vi "roller.vi"   [LabVIEW 2011]
uses:
  roller_internal_state.ctl
  roller_user_state.ctl
  signals/Signal.ctl
  roller_output_state.ctl
  roller_globals.vi
types:
  T1 = typedef "roller_internal_state.ctl" = enum16{"idle", "bump", "full", "fire_intermediate", "fire_finish", "fire_entry", "fire_end", "fire_recover"}
  T2 = typedef "WPI_DigitalInputDevRef.ctl" = cluster{"DevStatus":errorcluster, "DIO Channel":T3, "Digital Module":T4}
  T3 = typedef "FPGA_DIOChannel.ctl" = enum8{"DIO 1", "DIO 2", "DIO 3", "DIO 4", "DIO 5", "DIO 6", "DIO 7", "DIO 8", "DIO 9", "DIO 10", "DIO 11", "DIO 12", "DIO 13", "DIO 14", "Invalid"}
  T4 = typedef "FPGA_TypedefDigitalModule.ctl" = enum16{"Digital Module 1", "Digital Module 2"}
  T5 = typedef "WPI_MotorControlDeviceRef.ctl" = cluster{"DeviceStatus":errorcluster, "Type":enum16{"PWM", "CAN"}, "PWM":cluster{"Digital Module":T4, "PWM Channel":T6, "DeadBand":T7}, "CAN":cluster{"Device Number":u8, "Control Mode":T8, "Semaphore":T9, "Max Vout":dbl}, "Invert":bool, "TransformRef":T10, "InvTransformRef":T10}
  T6 = typedef "FPGA_DIOPWMChannel.ctl" = enum8{"PWM 1", "PWM 2", "PWM 3", "PWM 4", "PWM 5", "PWM 6", "PWM 7", "PWM 8", "PWM 9", "PWM 10", "Invalid"}
  T7 = typedef "WPI_PWMDeadband.ctl" = cluster{"Name":string, "maxPositivePwm":i32, "minPositivePwm":i32, "centerPwm":i32, "maxNegativePwm":i32, "minNegativePwm":i32, "angularRange":u16}
  T8 = typedef "WPI_CANJaguar_ControlMode.ctl" = enum8{"Percent VBus", "Current", "Speed", "Position", "Voltage"}
  T9 = typedef "Semaphore RefNum" = refnum<k1>
  T10 = typedef "WPI_PWMTransform_ConPane.ctl" = refnum<vi>
  T11 = cluster{"DigitalInputDevRef":T2, "DigitalInputDevRef":T2, "DigitalInputDevRef":T2, "DigitalInputDevRef":T2, "DigitalInputDevRef":T2}
  T12 = typedef "roller_user_state.ctl" = enum16{"off", "collect", "blow", "force suck"}
  T13 = cluster{"roller internal state":T1, "roller user state":T12, "sws":cluster{"r_sw_b1":bool, "r_sw_b2":bool, "r_sw_b3":bool, "r_sw_gun":bool, "r_sw_low":bool}}
  T14 = enum16{"push_data", "write_joe_johnson", "write_roller", "write_drivetrain", "write_gun_fast", "write_gun_slow"}
  T15 = typedef "Signal.ctl" = enum16{"SIGFIRE", "SIGSTOPSCRIPT", "SIGSTARTGUN", "SIGSTOPGUN", "SIGDISABLED", "SIGENABLED", "SIGUDPTIMEOUT", "SIGNEWVISION_REMOTE", "SIGNEWVISION_LOCAL", "SIGSHOTFIRED", "SIGDOTRACK", "SIGDONTTRACK"}
  T16 = typedef "roller_output_state.ctl" = enum16{"off", "suck", "blow"}
  T17 = cluster{"r_sw_b1":bool, "r_sw_b2":bool, "r_sw_b3":bool, "r_sw_gun":bool, "r_sw_low":bool}
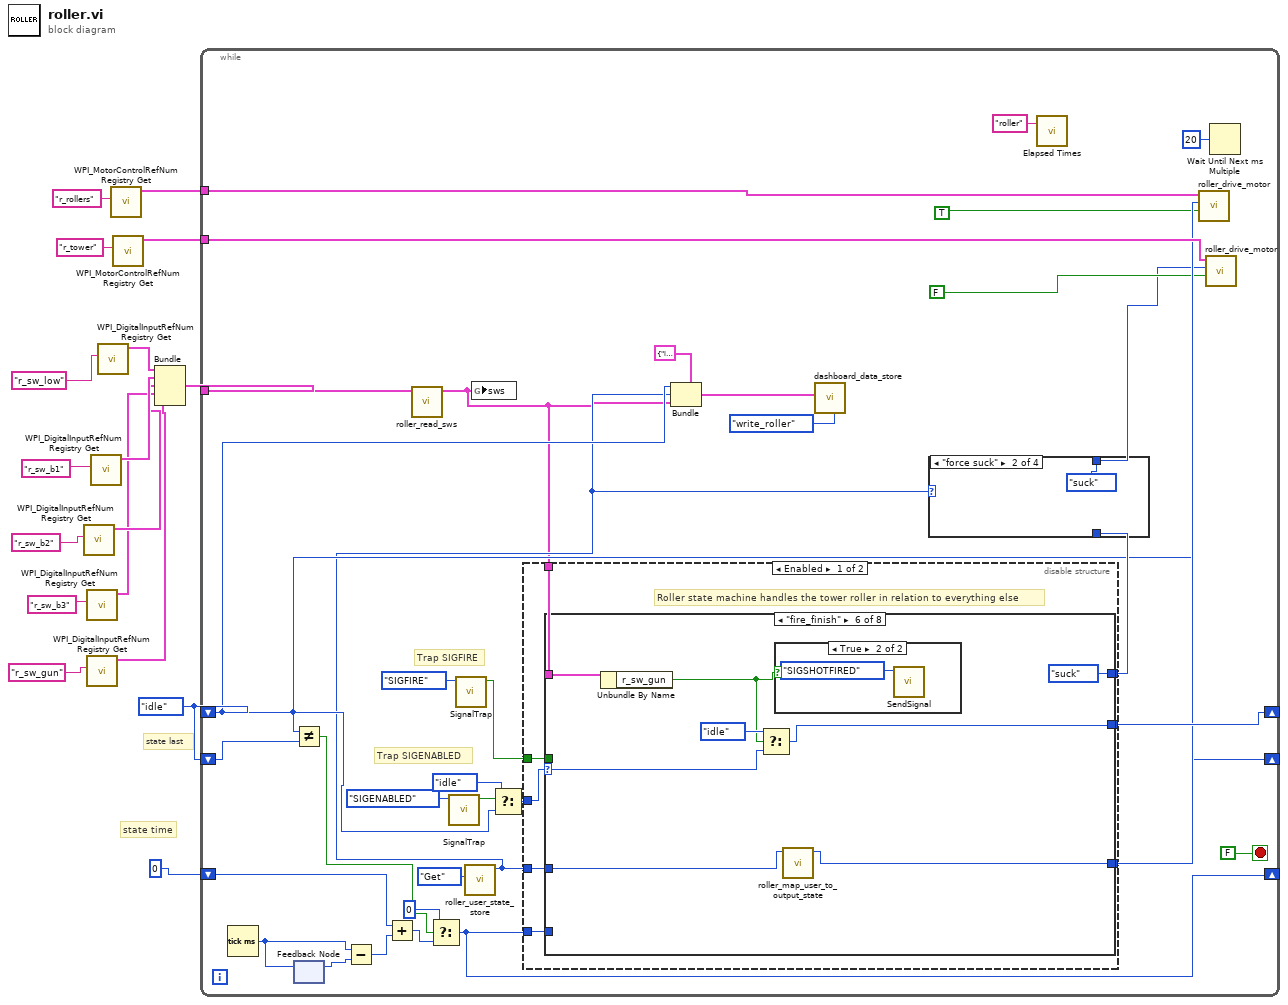
[diagram p0: block diagram]
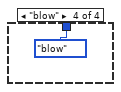
[diagram p4: hidden frame]
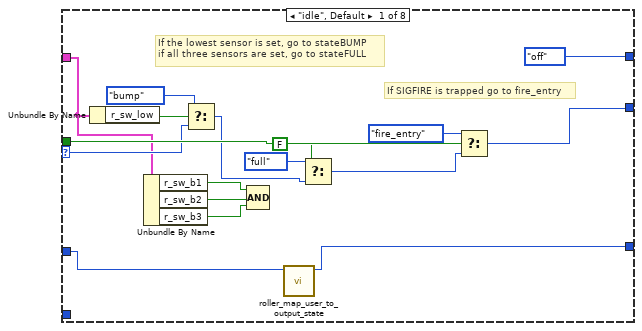
[diagram p5: hidden frame]
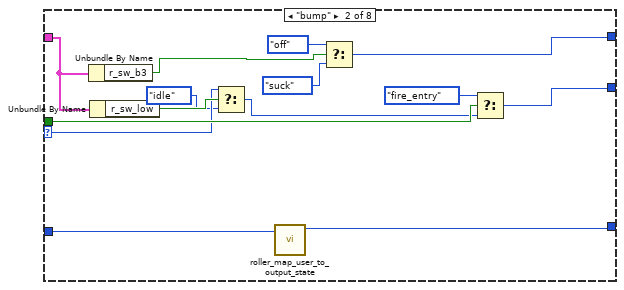
[diagram p6: hidden frame]
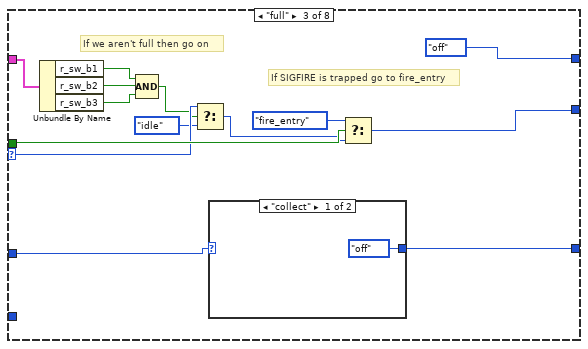
[diagram p7: hidden frame]
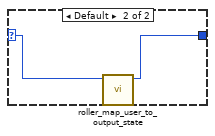
[diagram p8: hidden frame]
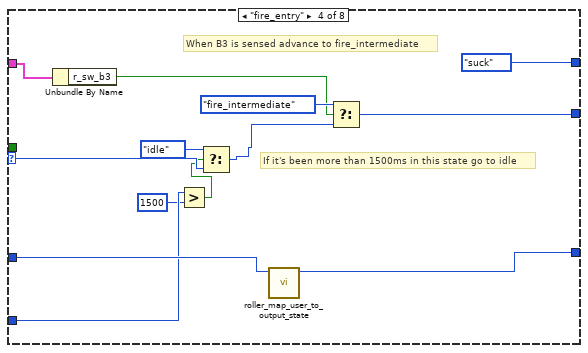
[diagram p9: hidden frame]
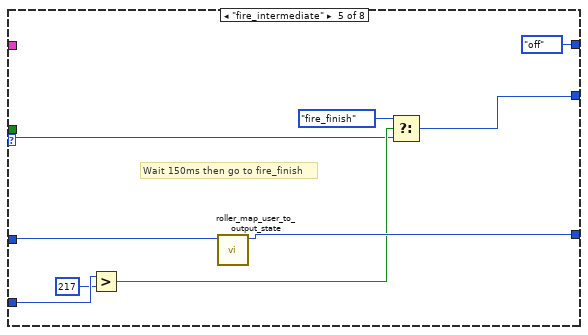
[diagram p10: hidden frame]
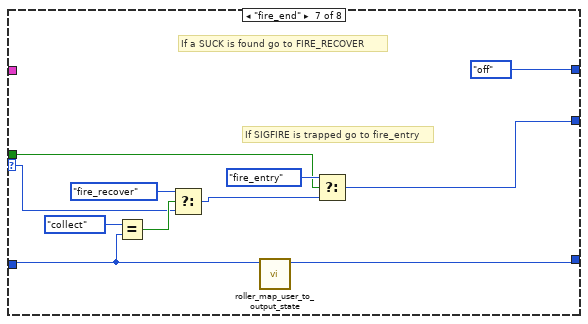
[diagram p12: hidden frame]
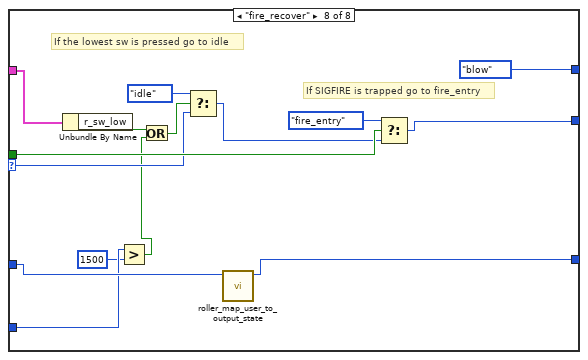
[diagram p13: hidden frame]
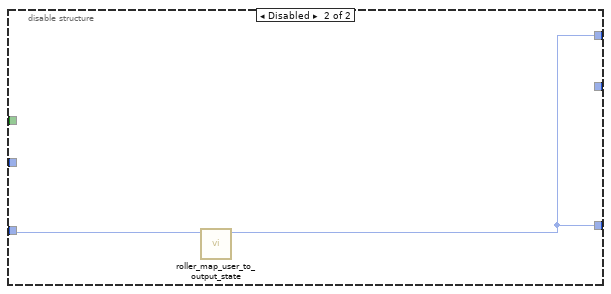
[diagram p14: hidden frame]
diagram:
  w1 = roller_internal_state."idle" ("roller internal state")
  # "state last"
  # "state time"
  n1 = call <vilib>:"WPI_DigitalInputRefNum Registry Get.vi"("refnum name"="r_sw_b2") -> ("DigitalInputDevRef"=w6:T2)  [unwired: 9 in, 1 out]
  n2 = call <vilib>:"WPI_DigitalInputRefNum Registry Get.vi"("refnum name"="r_sw_b3") -> ("DigitalInputDevRef"=w5:T2)  [unwired: 9 in, 1 out]
  n3 = call <vilib>:"WPI_DigitalInputRefNum Registry Get.vi"("refnum name"="r_sw_gun") -> ("DigitalInputDevRef"=w4:T2)  [unwired: 9 in, 1 out]
  n4 = call <vilib>:"WPI_DigitalInputRefNum Registry Get.vi"("refnum name"="r_sw_b1") -> ("DigitalInputDevRef"=w7:T2)  [unwired: 9 in, 1 out]
  n5 = call <vilib>:"WPI_DigitalInputRefNum Registry Get.vi"("refnum name"="r_sw_low") -> ("DigitalInputDevRef"=w8:T2)  [unwired: 9 in, 1 out]
  n6 = call <vilib>:"WPI_MotorControlRefNum Registry Get.vi"("refnum name"="r_rollers") -> ("MotorControlDevRef"=w15:T5)  [unwired: 9 in, 1 out]
  n7 = call <vilib>:"WPI_MotorControlRefNum Registry Get.vi"("refnum name"="r_tower") -> ("MotorControlDevRef"=w14:T5)  [unwired: 9 in, 1 out]
  n8 = Bundle("DigitalInputDevRef"=w8, "DigitalInputDevRef"=w7, "DigitalInputDevRef"=w6, "DigitalInputDevRef"=w5, "DigitalInputDevRef"=w4) -> (w3:T11)  [unwired: 1 in]
  n9 = while {
    tunnel: w15 -> [w49]
    tunnel: w14 -> [w48]
    tunnel: w3 -> [w47]
    shift-right: [w45] -> _
    shift-left: w1 -> [w20]
    shift-right: [w26] -> _
    shift-left: 0 -> [w30]
    shift-right: [w20] -> _
    shift-left: w1 -> [w32]
    stop <- FALSE stop-if-true
    # "Trap SIGENABLED"
    # "Trap SIGFIRE"
    n10 = Tick Count (ms)() -> (millisecond timer value=w33:u32)
    n11 = Not Equal?(x=w20, y=w32) -> (x != y?=w29:bool)
    n12 = feedback-in #1(w33) -> ()
    n13 = feedback #1() -> (w34:u32)  [unwired: 1 in]
    n14 = Subtract(x=w33, y=w34) -> (x-y=w31:u32)
    n15 = Add(x=w30, y=w31) -> (x+y=w28:u32)
    n16 = call "roller_read_sws.vi"("output cluster"=w47) -> ("sws"=w18:T17)  [unwired: 10 in]
    n17 = Select(t=u32 0, s=w29, f=w28) -> (s? t:f=w26:u32)
    n18 = call "SignalTrap.vi"("Signal"=Signal."SIGENABLED") -> ("Trapped Signal"=w37:bool)  [unwired: 10 in]
    n19 = call "SignalTrap.vi"("Signal"=Signal."SIGFIRE") -> ("Trapped Signal"=w44:bool)  [unwired: 10 in]
    n20 = call "roller_user_state_store.vi"("data_store_mode"=enum16{"Set", "Get"}."Get") -> ("roller user state out"=w19:T12)  [unwired: 10 in]
    n21 = global write "roller_globals.vi" "sws"(w18) -> ()
    n22 = Select(t=roller_internal_state."idle", s=w37, f=w20) -> (s? t:f=w36:T1)
    n23 = disable-structure shown="Enabled" {
      disable-tunnel: [w57 _] -> w45
      disable-tunnel: w44 -> [w63 _]
      disable-tunnel: [w62 w169] -> w24
      disable-tunnel: [w56 w169] -> w43
      disable-tunnel: w19 -> [w61 w170]
      disable-tunnel: w18 -> [w60 _]
      disable-tunnel: w36 -> [w59 _]
      disable-tunnel: w26 -> [w58 _]
      frame Enabled {
        # "Roller state machine handles the tower roller in relation to everything else"
        n24 = case shown="\"fire_finish\"" w59 {
          selector: w59 -> [w73 w88 w102 w116 w127 w137 w145 w162]
          tunnel: w63 -> [w80 w93 w107 _ _ _ w152 w167]
          tunnel: [roller_output_state."off" ("roller output state") w81 roller_output_state."off" ("roller output state") roller_output_state."suck" ("roller output state") roller_output_state."off" ("roller output state") roller_output_state."suck" ("roller output state") roller_output_state."off" ("roller output state") roller_output_state."blow" ("roller output state")] -> w62
          tunnel: w61 -> [w77 w91 w95 w124 w130 w141 w148 w165]
          tunnel: w60 -> [w71 w85 w100 w121 _ w138 _ w160]
          tunnel: w58 -> [_ _ _ w115 w132 _ _ w156]
          tunnel: [w78 w92 w106 w119 w126 w136 w151 w166] -> w57
          tunnel: [w76 w90 w104 w123 w129 w140 w150 w164] -> w56
          frame "idle", Default {
            # "If the lowest sensor is set, go to stateBUMP\nif all three sensors are set, go to stateFULL"
            # "If SIGFIRE is trapped go to fire_entry"
            n25 = Unbundle By Name(w71) -> ("r_sw_low"=w74:bool)
            n26 = Unbundle By Name(w71) -> ("r_sw_b1"=w70:bool, "r_sw_b2"=w69:bool, "r_sw_b3"=w68:bool)
            n27 = Select(t=roller_internal_state."bump", s=w74, f=w73) -> (s? t:f=w67:T1)
            n28 = Compound Arithmetic op=AND(w70, w69, w68) -> ()  [unwired: 1 out]
            n29 = call "roller_map_user_to_output_state.vi"("roller user state"=w77) -> ("roller output state"=w76:T16)  [unwired: 10 in]
            n30 = Select(t=roller_internal_state."full", s=FALSE, f=w67) -> (s? t:f=w65:T1)
            n31 = Select(t=roller_internal_state."fire_entry", s=w80, f=w65) -> (s? t:f=w78:T1)
          }
          frame "bump" {
            n32 = Unbundle By Name(w85) -> ("r_sw_b3"=w82:bool)
            n33 = Unbundle By Name(w85) -> ("r_sw_low"=w89:bool)
            n34 = Select(t=w88, s=w89, f=roller_internal_state."idle") -> (s? t:f=w86:T1)
            n35 = call "roller_map_user_to_output_state.vi"("roller user state"=w91) -> ("roller output state"=w90:T16)  [unwired: 10 in]
            n36 = Select(t=roller_output_state."off", s=w82, f=roller_output_state."suck" ("roller output state")) -> (s? t:f=w81:T16)
            n37 = Select(t=roller_internal_state."fire_entry", s=w93, f=w86) -> (s? t:f=w92:T1)
          }
          frame "full" {
            # "If we aren't full then go on"
            # "If SIGFIRE is trapped go to fire_entry"
            n38 = Unbundle By Name(w100) -> ("r_sw_b1"=w99:bool, "r_sw_b2"=w98:bool, "r_sw_b3"=w97:bool)
            n39 = Compound Arithmetic op=AND(w99, w98, w97) -> (w96:bool)
            n40 = Select(t=w102, s=w96, f=roller_internal_state."idle") -> (s? t:f=w103:T1)
            n41 = case shown="\"collect\"" w95 {
              selector: w95 -> [_ w110]
              tunnel: [roller_output_state."off" ("roller output state") w111] -> w104
              frame "collect" {
              }
              frame Default {
                n42 = call "roller_map_user_to_output_state.vi"("roller user state"=w110) -> ("roller output state"=w111:T16)  [unwired: 10 in]
              }
            }
            n43 = Select(t=roller_internal_state."fire_entry", s=w107, f=w103) -> (s? t:f=w106:T1)
          }
          frame "fire_entry" {
            # "If it's been more than 1500ms in this state go to idle"
            # "When B3 is sensed advance to fire_intermediate"
            n44 = Unbundle By Name(w121) -> ("r_sw_b3"=w120:bool)
            n45 = Greater?(x=w115, y=u32 1500) -> (0:w113:bool)
            n46 = Select(t=roller_internal_state."idle", s=w113, f=w116) -> (s? t:f=w117:T1)
            n47 = call "roller_map_user_to_output_state.vi"("roller user state"=w124) -> ("roller output state"=w123:T16)  [unwired: 10 in]
            n48 = Select(t=roller_internal_state."fire_intermediate", s=w120, f=w117) -> (s? t:f=w119:T1)
          }
          frame "fire_intermediate" {
            # "Wait 150ms then go to fire_finish"
            n49 = Greater?(x=w132, y=u32 217) -> (0:w128:bool)
            n50 = call "roller_map_user_to_output_state.vi"("roller user state"=w130) -> ("roller output state"=w129:T16)  [unwired: 10 in]
            n51 = Select(t=roller_internal_state."fire_finish", s=w128, f=w127) -> (s? t:f=w126:T1)
          }
          frame "fire_finish" {
            n52 = Unbundle By Name(w138) -> ("r_sw_gun"=w134:bool)
            n53 = Select(t=roller_internal_state."idle", s=w134, f=w137) -> (s? t:f=w136:T1)
            n54 = case shown="True" w134 {
              frame False {
              }
              frame True {
                n55 = call "SendSignal.vi"("Signal"=Signal."SIGSHOTFIRED") -> ()  [unwired: 11 in]
              }
            }
            n56 = call "roller_map_user_to_output_state.vi"("roller user state"=w141) -> ("roller output state"=w140:T16)  [unwired: 10 in]
          }
          frame "fire_end" {
            # "If a SUCK is found go to FIRE_RECOVER"
            # "If SIGFIRE is trapped go to fire_entry"
            n57 = Equal?(x=roller_user_state."collect", y=w148) -> (x = y?=w146:bool)
            n58 = Select(t=roller_internal_state."fire_recover", s=w146, f=w145) -> (s? t:f=w144:T1)
            n59 = call "roller_map_user_to_output_state.vi"("roller user state"=w148) -> ("roller output state"=w150:T16)  [unwired: 10 in]
            n60 = Select(t=roller_internal_state."fire_entry", s=w152, f=w144) -> (s? t:f=w151:T1)
          }
          frame "fire_recover" {
            # "If the lowest sw is pressed go to idle"
            # "If SIGFIRE is trapped go to fire_entry"
            n61 = Unbundle By Name(w160) -> ("r_sw_low"=w158:bool)
            n62 = Greater?(x=w156, y=u32 1500) -> (0:w155:bool)
            n63 = Or(x=w158, y=w155) -> (x .or. y?=w157:bool)
            n64 = Select(t=roller_internal_state."idle", s=w157, f=w162) -> (s? t:f=w163:T1)
            n65 = call "roller_map_user_to_output_state.vi"("roller user state"=w165) -> ("roller output state"=w164:T16)  [unwired: 10 in]
            n66 = Select(t=roller_internal_state."fire_entry", s=w167, f=w163) -> (s? t:f=w166:T1)
          }
        }
      }
      frame Disabled {
        n67 = call "roller_map_user_to_output_state.vi"("roller user state"=w170) -> ("roller output state"=w169:T16)  [unwired: 10 in]
      }
    }
    n68 = Bundle(cluster=T13 {"roller internal state"=enum."idle", "roller user state"=enum."off", "sws"={"r_sw_b1"=FALSE, "r_sw_b2"=FALSE, "r_sw_b3"=FALSE, "r_sw_gun"=FALSE, "r_sw_low"=FALSE}} ("roller data"), "roller internal state"=w20, "roller user state"=w19, "sws"=w18) -> (w21:T13)
    n69 = call "dashboard_data_store.vi"("mode"=T14."write_roller", "roller data"=w21) -> ()  [unwired: 10 in]
    n70 = case shown="\"force suck\"" w19 {
      tunnel: [w52 roller_output_state."suck" ("roller output state") w54 roller_output_state."blow" ("roller output state")] -> w25
      tunnel: w24 -> [w52 _ w54 _]
      frame "off", Default {
      }
      frame "force suck" {
      }
      frame "collect" {
      }
      frame "blow" {
      }
    }
    n71 = call "Elapsed Times.vi"("Call Name"="roller") -> ()  [unwired: 2 in, 1 out]
    n72 = call "roller_drive_motor.vi"("invert"=TRUE, "roller output state"=w43, "MotorControlDevRef"=w49) -> ()  [unwired: 9 in]
    n73 = call "roller_drive_motor.vi"("invert"=FALSE, "roller output state"=w25, "MotorControlDevRef"=w48) -> ()  [unwired: 9 in]
    n74 = Wait Until Next ms Multiple(millisecond multiple=u32 20) -> ()  [unwired: 1 out]
  }
